vi "Get Run Number.vi"() -> (1 "Run Number":i32)   [LabVIEW 2026, in "TALOS.lvlib"]
uses:
  TALOS.lvlib
  Global Memory.vi
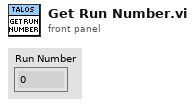
[diagram p1: front panel]
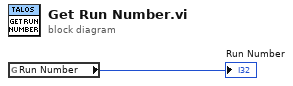
[diagram p0: block diagram]
diagram:
  n1 = global read "Global Memory.vi" "Run Number"() -> (→"Run Number":i32)
